vi "From Pythonic - Float Array.vi"(4 "Pythonic Value":string) -> (1 "Float Array":dbl[](array[numeric]))   [LabVIEW 2012, in "OPI.lvclass"]
doc: "Convert pythonic values into LabVIEW data. This method can be helpfull to convert elements of tuples or dictionaries.\n\nReturn a 1D array of float - LabVIEW Double representation."
uses:
  OPI.lvclass
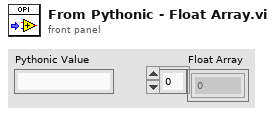
[diagram p1: front panel]
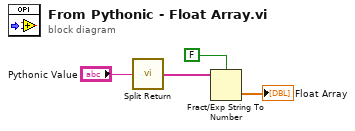
[diagram p0: block diagram]
diagram:
  n1 = call "Split Return.vi"("Return Value"="Pythonic Value") -> ("Split String"=w4:string[])
  n2 = Fract/Exp String To Number(use system decimal point (T)=FALSE, string=w4) -> (number=→"Float Array":dbl[])  [unwired: 2 in, 1 out]
